vi "SortArray.vi"(11 "Input Array":string[](array[string])) -> (3 "Output Array":string[](array[string]))   [LabVIEW 2019, in "ArrayUtilities.lvlib"]
uses:
  ArrayUtilities.lvlib
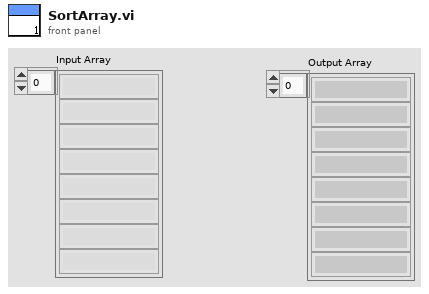
[diagram p1: front panel]
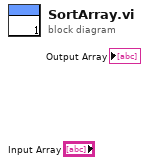
[diagram p0: block diagram]
diagram:
